vi "Digital_Timer.vi"(1 "Start_Time":timestamp, 2 "Current_Time":timestamp) -> (0 "Timer_Out":string)   [LabVIEW 2016]
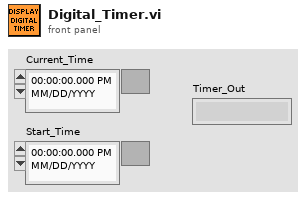
[diagram p1: front panel]
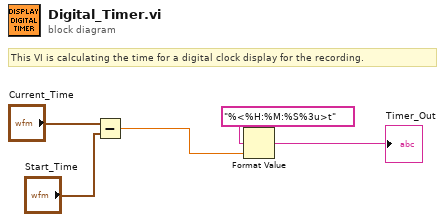
[diagram p0: block diagram]
diagram:
  # "This VI is calculating the time for a digital clock display for the recording."
  n1 = Subtract(x="Current_Time", y="Start_Time") -> (x-y=w3:dbl)
  n2 = Format Value(format string="%<%H:%M:%S%3u>t", value (0)=w3) -> (output string=→"Timer_Out":string)  [unwired: 1 in]
